vi "PRAT Solenoid.vi"(0 "VISA session":refnum<visa-resource-name>="MW100", 5 "PRAT Channels":T2, 7 "Normally Open Valve":T1, 11 "Error In":errorcluster) -> (4 "dup VISA session":refnum<visa-resource-name>, 15 "Error Out":errorcluster)   [LabVIEW 2016]
uses:
  Type Definitions/PRAT Channel Settings.ctl
  Type Definitions/HEWH Normally Open Valve Control.ctl
panel:
  out "Retries":i32
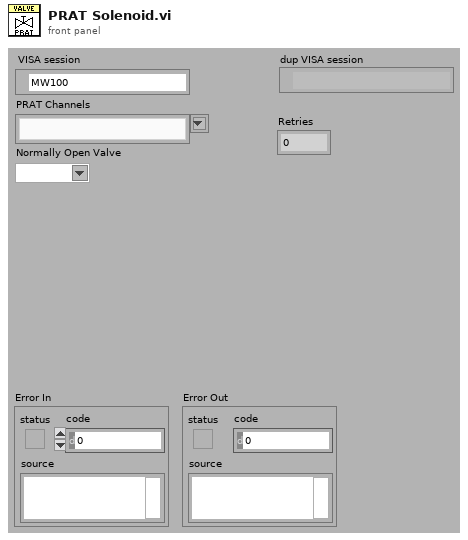
[diagram p1: front panel]
types:
  T1 = typedef "HEWH Normally Open Valve Control.ctl" = string
  T2 = typedef "PRAT Channel Settings.ctl" = string
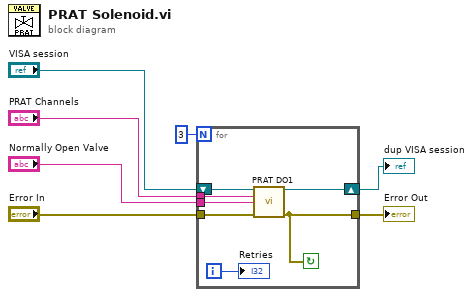
[diagram p0: block diagram]
diagram:
  n1 = for {
    N: 3 -> [_]
    tunnel: "PRAT Channels" -> [w13]
    shift-right: [w12] -> w5
    shift-left: "VISA session" -> [w14]
    tunnel: "Error In" -> [w10]
    tunnel: [w9] -> w2
    tunnel: "Normally Open Valve" -> [w8]
    i -> [w11]
    stop <- w9 continue-if-true
    n2 = call "PRAT DO1.vi"("VISA session"=w14, "PRAT Channels"=w13, "Normally Open Valve"=w8, "Error In"=w10) -> ("dup VISA session"=w12:refnum<visa-resource-name>, "error out"=w9:errorcluster)  [unwired: 10 in]
    "Retries" <- w11
  }
  "Error Out" <- w2
  "dup VISA session" <- w5
